vi "Read new data.vi"(7 "Scope":T1={"Config"={"VISA Resource"="", "Model"=enum."DPO 3012", "Timebase"=0.0, "Timeout (ms)"=0, "TAS"={"Vertical Range (V)"=0.0, "Vertical Offset (0.0 divs)"=0.0, "Bandwidth"=0, "Probe Attenuation (10.0)"=0.0, "Vertical Coupling"=0, "Impedance"=0, "Multiplication factor"=0.0, "Channel"=enum."Channel 1"}, "TPC"={"Vertical Range (V)"=0.0, "Vertical Offset (0.0 divs)"=0.0, "Bandwidth"=0, "Probe Attenuation (10.0)"=0.0, "Vertical Coupling"=0, "Impedance"=0, "Multiplication factor"=0.0, "Channel"=enum."Channel 1"}, "Trigger"={"Mode"=enum."Laser (TAS)", "Source "=enum."Channel 1", "PIA"={"Test LEDs"=FALSE, "LED line"="", "LED off (s)"=0.0, "LED on (s)"=0.0}, "Threshold (V)"=0.0004}}, "Indicators"={"Setup"={"Final number of points"=0.0, "Pretrigger points"=0.0, "Number of readouts"=0, "Model"={"Acquisition Type"=0, "Record length (points)"=0, "Averages on scope"=0, "Average number of points"=0.0}}, "Timestamp of Data"=timestamp(0 s since 1904-01-01)}, "Data"={"TPC"={"Live data"={"t0"=timestamp(0 s since 1904-01-01), "dt"=1.0, "Y"=[]}, "Averaged data"={"t0"=timestamp(0 s since 1904-01-01), "dt"=1.0, "Y"=[]}, "Accumulated data"={"t0"=timestamp(0 s since 1904-01-01), "dt"=1.0, "Y"=[]}, "Final data"={"t0"=timestamp(0 s since 1904-01-01), "dt"=1.0, "Y"=[]}}, "TAS"={"Live data"={"t0"=timestamp(0 s since 1904-01-01), "dt"=1.0, "Y"=[]}, "Averaged data"={"t0"=timestamp(0 s since 1904-01-01), "dt"=1.0, "Y"=[]}, "Accumulated data"={"t0"=timestamp(0 s since 1904-01-01), "dt"=1.0, "Y"=[]}, "Final data"={"t0"=timestamp(0 s since 1904-01-01), "dt"=1.0, "Y"=[]}}, "Time arrays"={"Time array (decimated)"=[], "waveform"={"t0"=timestamp(0 s since 1904-01-01), "dt"=1.0, "Y"=[]}}}, "Test"={"Config"={"Amplification Factor"=2.0, "100% Reflectance Standard"=2.0, "Calculation Method"=enum."Reflectance", "Option to discard new data?"=FALSE, "Mode"=enum."Spectrum", "Number of Averages"=0, "B Test?"=FALSE}, "Indicators"={"DAQ Background Level (V)"=2.0, "A-Test Counter"=2, "B-Test Counter"=2, "Type"=enum."A-Test", "Scope Background Level (Amps)"=2.0, "TAS only?"=FALSE}}} {"Test"."Config"."Number of Averages" min=0; "Indicators"."Setup"."Model"."Record length (points)" items=["1000"=1, "10,000"=10, "100,000"=100, "1,000,000"=1000, "5,000,000"=5000, "10,000,000"=10000]; "Indicators"."Setup"."Model"."Acquisition Type" items=["Sample", "Peak Detect", "Hi Res", "Envelope", "Average"]; "Config"."Trigger"."Threshold (V)" format="%#_3f"; "Config"."TPC"."Impedance" items=["1M", "75", "50"]; "Config"."TPC"."Vertical Coupling" items=["AC", "DC", "Ground"]; "Config"."TPC"."Bandwidth" items=["FULL", "250 MHz", "150 MHz", "20 MHz"]; "Config"."TAS"."Impedance" items=["1M", "75", "50"]; "Config"."TAS"."Vertical Coupling" items=["AC", "DC", "Ground"]; "Config"."TAS"."Bandwidth" items=["FULL", "250 MHz", "150 MHz", "20 MHz"]; "Config"."Timebase" format="%^#_3e"}, 8 "error in (no error)":errorcluster) -> (0 "error out":errorcluster, 3 "Two channels read":bool=TRUE, 5 "Scope out":T1={"Config"={"VISA Resource"="", "Model"=enum."DPO 3012", "Timebase"=0.0, "Timeout (ms)"=0, "TAS"={"Vertical Range (V)"=0.0, "Vertical Offset (0.0 divs)"=0.0, "Bandwidth"=0, "Probe Attenuation (10.0)"=0.0, "Vertical Coupling"=0, "Impedance"=0, "Multiplication factor"=0.0, "Channel"=enum."Channel 1"}, "TPC"={"Vertical Range (V)"=0.0, "Vertical Offset (0.0 divs)"=0.0, "Bandwidth"=0, "Probe Attenuation (10.0)"=0.0, "Vertical Coupling"=0, "Impedance"=0, "Multiplication factor"=0.0, "Channel"=enum."Channel 1"}, "Trigger"={"Mode"=enum."Laser (TAS)", "Source "=enum."Channel 1", "PIA"={"Test LEDs"=FALSE, "LED line"="", "LED off (s)"=0.0, "LED on (s)"=0.0}, "Threshold (V)"=0.0004}}, "Indicators"={"Setup"={"Final number of points"=0.0, "Pretrigger points"=0.0, "Number of readouts"=0, "Model"={"Acquisition Type"=0, "Record length (points)"=0, "Averages on scope"=0, "Average number of points"=0.0}}, "Timestamp of Data"=timestamp(0 s since 1904-01-01)}, "Data"={"TPC"={"Live data"={"t0"=timestamp(0 s since 1904-01-01), "dt"=1.0, "Y"=[]}, "Averaged data"={"t0"=timestamp(0 s since 1904-01-01), "dt"=1.0, "Y"=[]}, "Accumulated data"={"t0"=timestamp(0 s since 1904-01-01), "dt"=1.0, "Y"=[]}, "Final data"={"t0"=timestamp(0 s since 1904-01-01), "dt"=1.0, "Y"=[]}}, "TAS"={"Live data"={"t0"=timestamp(0 s since 1904-01-01), "dt"=1.0, "Y"=[]}, "Averaged data"={"t0"=timestamp(0 s since 1904-01-01), "dt"=1.0, "Y"=[]}, "Accumulated data"={"t0"=timestamp(0 s since 1904-01-01), "dt"=1.0, "Y"=[]}, "Final data"={"t0"=timestamp(0 s since 1904-01-01), "dt"=1.0, "Y"=[]}}, "Time arrays"={"Time array (decimated)"=[], "waveform"={"t0"=timestamp(0 s since 1904-01-01), "dt"=1.0, "Y"=[]}}}, "Test"={"Config"={"Amplification Factor"=2.0, "100% Reflectance Standard"=2.0, "Calculation Method"=enum."Reflectance", "Option to discard new data?"=FALSE, "Mode"=enum."Spectrum", "Number of Averages"=0, "B Test?"=FALSE}, "Indicators"={"DAQ Background Level (V)"=2.0, "A-Test Counter"=2, "B-Test Counter"=2, "Type"=enum."A-Test", "Scope Background Level (Amps)"=2.0, "TAS only?"=FALSE}}} {"Test"."Config"."Number of Averages" min=0; "Indicators"."Setup"."Model"."Record length (points)" items=["1000"=1, "10,000"=10, "100,000"=100, "1,000,000"=1000, "5,000,000"=5000, "10,000,000"=10000]; "Indicators"."Setup"."Model"."Acquisition Type" items=["Sample", "Peak Detect", "Hi Res", "Envelope", "Average"]; "Config"."Trigger"."Threshold (V)" format="%#_3f"; "Config"."TPC"."Impedance" items=["1M", "75", "50"]; "Config"."TPC"."Vertical Coupling" items=["AC", "DC", "Ground"]; "Config"."TPC"."Bandwidth" items=["FULL", "250 MHz", "150 MHz", "20 MHz"]; "Config"."TAS"."Impedance" items=["1M", "75", "50"]; "Config"."TAS"."Vertical Coupling" items=["AC", "DC", "Ground"]; "Config"."TAS"."Bandwidth" items=["FULL", "250 MHz", "150 MHz", "20 MHz"]; "Config"."Timebase" format="%^#_3e"})   [LabVIEW 2017, in "Scope.lvlib"]
doc: "Acquires either two channels or one channel of data from the scope, \ndepending on the mode (B-test only acquires Ch1/TAS data) and the \nuser's TPC channel selection (if channel is \"None\", we shouldn't acquire \ndata from it)"
uses:
  Scope.lvlib
  Controls/Params.ctl
  Controls/Models.ctl
  Controls/TPC.ctl
  Controls/Channels.ctl
  Trigger/Controls/Params.ctl
  Trigger/Controls/Mode.ctl
  Trigger/Controls/Trigger channels.ctl
  Controls/Acquisition type.ctl
  Controls/Record length.ctl
  Controls/Data.ctl
  Controls/Channel data.ctl
  System Control/CTLs/Test params.ctl
  System Control/CTLs/Test Controls.ctl
  System Control/CTLs/Test indicators.ctl
  System Control/CTLs/Test Type.ctl
  <vilib>/Waveform/WDTOps.llb/WDT Index Channel DBL.vi
  <vilib>/Utility/error.llb/Error Cluster From Error Code.vi
  <vilib>/ErrorRing/Error Ring.xnode
  Third Party Drivers/Tektronix DPO MSO 2000 4000 Series/Tektronix DPO MSO 2000 4000 Series.lvlib
  Processing/Processing.lvlib
  Trigger/Trigger.lvlib
  System Control/Main controller.lvlib
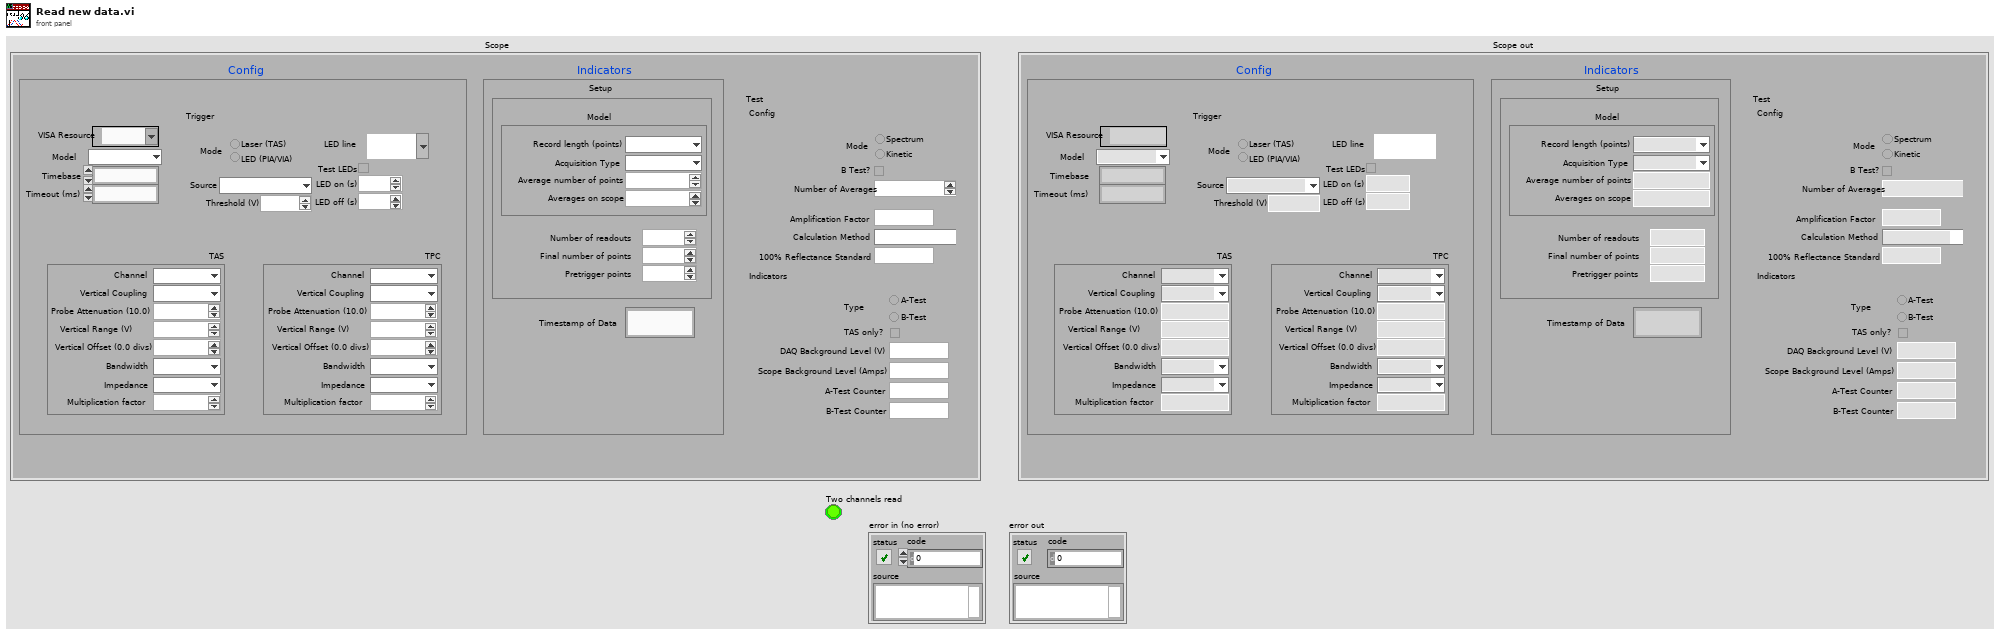
[diagram p1: front panel]
types:
  T1 = typedef "Scope.lvlib/Params.ctl" = cluster{"Config":cluster{"VISA Resource":refnum<visa-resource-name>, "Model":T2, "Timebase":dbl, "Timeout (ms)":u32, "TAS":T3, "TPC":T3, "Trigger":T5}, "Indicators":cluster{"Setup":cluster{"Final number of points":dbl, "Pretrigger points":dbl, "Number of readouts":i32, "Model":cluster{"Acquisition Type":T8, "Record length (points)":T9, "Averages on scope":i32, "Average number of points":dbl}}, "Timestamp of Data":timestamp}, "Data":T10, "Test":T12}
  T2 = typedef "Scope.lvlib/Models.ctl" = enum16{"DPO 3012", "DPO 2012B", "TDS 3012C"}
  T3 = typedef "Scope.lvlib/TPC.ctl" = cluster{"Vertical Range (V)":dbl, "Vertical Offset (0.0 divs)":dbl, "Bandwidth":i32, "Probe Attenuation (10.0)":dbl, "Vertical Coupling":u16, "Impedance":u16, "Multiplication factor":dbl, "Channel":T4}
  T4 = typedef "Scope.lvlib/Channels.ctl" = enum16{"Channel 1", "Channel 2", "Channel 3", "Channel 4", "Math", "Reference A", "Reference B", "Reference C", "Reference D", "B1", "B2", "None"}
  T5 = typedef "Scope.lvlib/Trigger.lvlib/Params.ctl" = cluster{"Mode":T6, "Source ":T7, "PIA":cluster{"Test LEDs":bool, "LED line":tag, "LED off (s)":dbl, "LED on (s)":dbl}, "Threshold (V)":dbl}
  T6 = typedef "Scope.lvlib/Trigger.lvlib/Mode.ctl" = enum32{"Laser (TAS)", "LED (PIA/VIA)"}
  T7 = typedef "Scope.lvlib/Trigger.lvlib/Trigger channels.ctl" = enum16{"Channel 1", "Channel 2", "Channel 3", "Channel 4", "AC Line", "Aux", "Digital Channel 0", "Digital Channel 1", "Digital Channel 2", "Digital Channel 3", "Digital Channel 4", "Digital Channel 5", "Digital Channel 6", "Digital Channel 7", "Digital Channel 8", "Digital Channel 9", "Digital Channel 10", "Digital Channel 11", "Digital Channel 12", "Digital Channel 13", "Digital Channel 14", "Digital Channel 15", "RF"}
  T8 = typedef "Scope.lvlib/Acquisition type.ctl" = u16
  T9 = typedef "Scope.lvlib/Record length.ctl" = u32
  T10 = typedef "Scope.lvlib/Data.ctl" = cluster{"TPC":T11, "TAS":T11, "Time arrays":cluster{"Time array (decimated)":dbl[], "waveform":waveform(dbl)}}
  T11 = typedef "Scope.lvlib/Channel data.ctl" = cluster{"Live data":waveform(dbl), "Averaged data":waveform(dbl), "Accumulated data":waveform(dbl), "Final data":waveform(dbl)}
  T12 = typedef "Main controller.lvlib/Test params.ctl" = cluster{"Config":T13, "Indicators":T14}
  T13 = typedef "Main controller.lvlib/Test Controls.ctl" = cluster{"Amplification Factor":dbl, "100% Reflectance Standard":dbl, "Calculation Method":enum16{"Reflectance", "Transmission", "Kubelka-Munk"}, "Option to discard new data?":bool, "Mode":enum32{"Spectrum", "Kinetic"}, "Number of Averages":i32, "B Test?":bool}
  T14 = typedef "Main controller.lvlib/Test indicators.ctl" = cluster{"DAQ Background Level (V)":dbl, "A-Test Counter":i32, "B-Test Counter":i32, "Type":T15, "Scope Background Level (Amps)":dbl, "TAS only?":bool}
  T15 = typedef "Main controller.lvlib/Test Type.ctl" = enum32{"A-Test", "B-Test"}
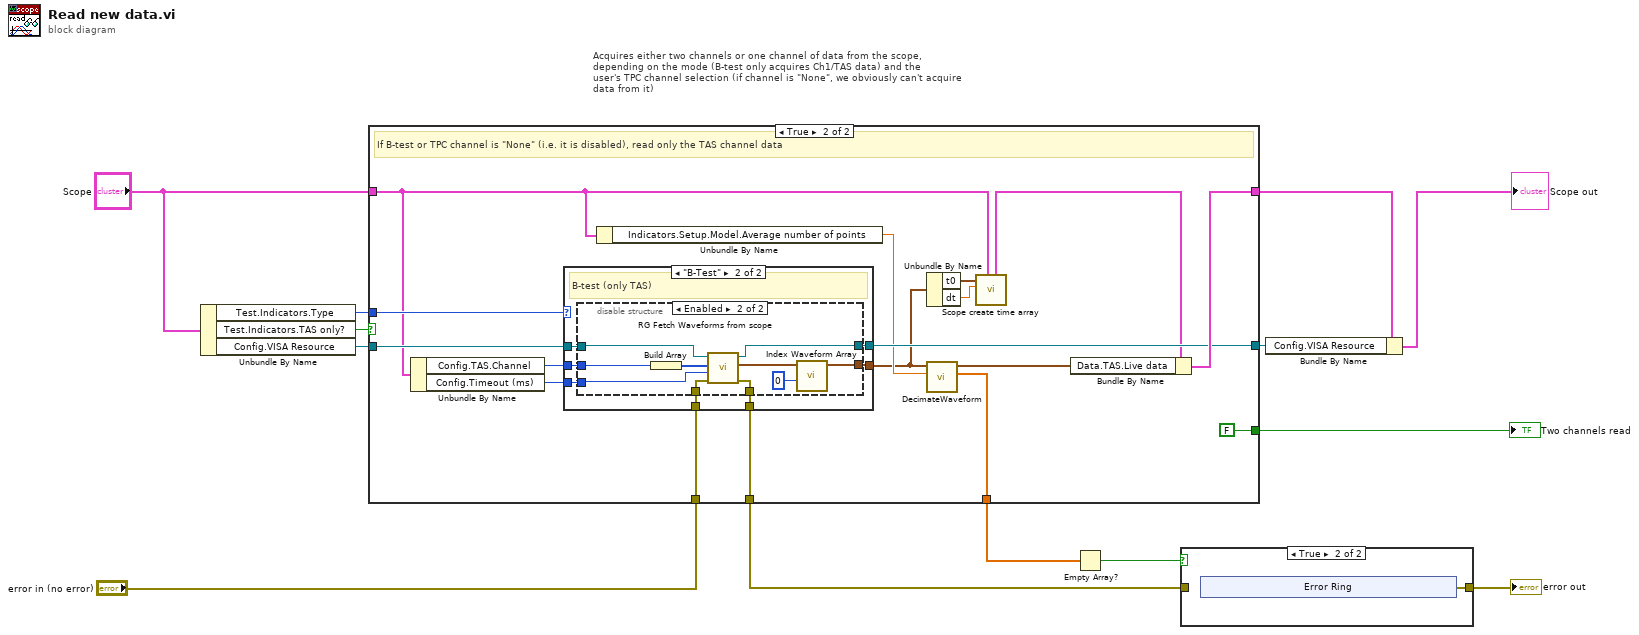
[diagram p0: block diagram]
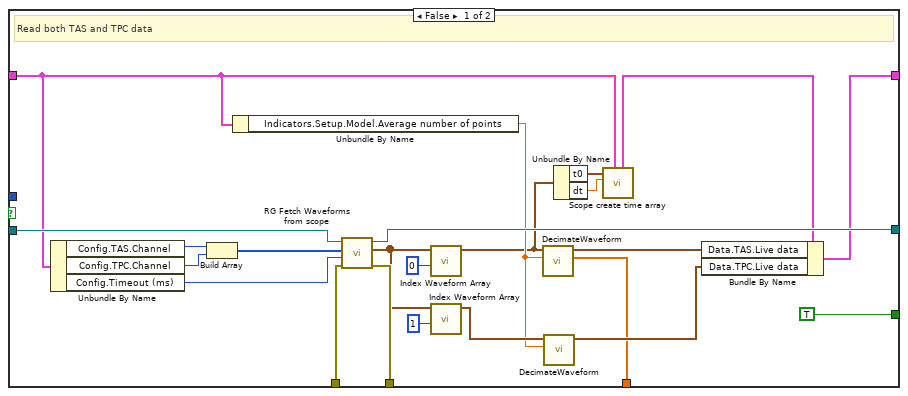
[diagram p2: hidden frame]
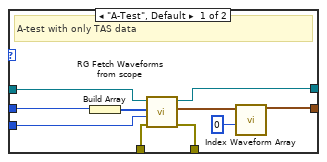
[diagram p3: hidden frame]
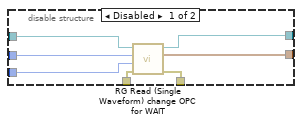
[diagram p4: hidden frame]
diagram:
  # "Acquires either two channels or one channel of data from the scope, \ndepending on the mode (B-test only acquires Ch1/TAS data) and the\nuser's TPC channel selection (if channel is \"None\", we obviously can't acquire data from it)"
  n1 = Unbundle By Name("Scope") -> ("Test.Indicators.Type"=w3:T15, "Test.Indicators.TAS only?"=w4:bool, "Config.VISA Resource"=w5:refnum<visa-resource-name>)
  n2 = case shown="True" w4 {
    tunnel: "error in (no error)" -> [w36 w50]
    tunnel: [w35 w49] -> w10
    tunnel: [w20 w42] -> w1
    tunnel: [w30 w51] -> w9
    tunnel: w5 -> [w29 w52]
    tunnel: "Scope" -> [w15 w41]
    tunnel: [w28 w53] -> w8
    tunnel: w3 -> [_ w46]
    tunnel: [TRUE FALSE] -> w6
    frame False {
      # "Read both TAS and TPC data"
      n3 = Unbundle By Name(w15) -> ("Config.TAS.Channel"=w33:T4, "Config.TPC.Channel"=w32:T4, "Config.Timeout (ms)"=w34:u32)
      n4 = Build Array(w33, w32) -> (w31:T4[])
      n5 = Unbundle By Name(w15) -> ("Indicators.Setup.Model.Average number of points"=w21:dbl)
      n6 = call "RG Fetch Waveforms from scope.vi"("error in (no error)"=w36, "Maximum Time (10000ms)"=w34, "Channels"=w31, "VISA resource name"=w29) -> ("error out"=w35:errorcluster, "Waveform Data"=w19:waveform(dbl)[], "VISA resource name out"=w30:refnum<visa-resource-name>)  [unwired: 5 in]
      n7 = call-poly <vilib>:"Index Waveform Array.vi"("index"=0, "waveform array"=w19) -> ("waveform"=w16:waveform(dbl))  [unwired: 8 in, 1 out]
      n8 = call-poly <vilib>:"Index Waveform Array.vi"("index"=1, "waveform array"=w19) -> ("waveform"=w23:waveform(dbl))  [unwired: 8 in, 1 out]
      n9 = call "DecimateWaveform.vi"("Decimating factor"=w21, "waveform in"=w16) -> ("Y"=w20:dbl[], "waveform out"=w22:waveform(dbl))  [unwired: 8 in]
      n10 = call "DecimateWaveform.vi"("Decimating factor"=w21, "waveform in"=w23) -> ("waveform out"=w24:waveform(dbl))  [unwired: 8 in, 1 out]
      n11 = Unbundle By Name(w16) -> ("t0"=w18:timestamp, "dt"=w17:dbl)
      n12 = call "Scope create time array.vi"("Scope"=w15, "dt"=w17, "t0"=w18) -> ("Scope Out"=w14:T1)  [unwired: 6 in, 2 out]
      n13 = Bundle By Name(cluster=w14, "Data.TAS.Live data"=w22, "Data.TPC.Live data"=w24) -> (w28:T1)
    }
    frame True {
      # "If B-test or TPC channel is \"None\" (i.e. it is disabled), read only the TAS channel data"
      n14 = Unbundle By Name(w41) -> ("Config.TAS.Channel"=w48:T4, "Config.Timeout (ms)"=w47:u32)
      n15 = case shown="\"B-Test\"" w46 {
        tunnel: w52 -> [w63 w67]
        tunnel: [w62 w68] -> w51
        tunnel: w50 -> [w60 w70]
        tunnel: [w59 w69] -> w49
        tunnel: w48 -> [w56 w66]
        tunnel: w47 -> [w61 w65]
        tunnel: [w57 w64] -> w39
        frame "A-Test", Default {
          # "A-test with only TAS data"
          n16 = Build Array(w56) -> (w55:T4[])
          n17 = call "RG Fetch Waveforms from scope.vi"("error in (no error)"=w60, "Maximum Time (10000ms)"=w61, "Channels"=w55, "VISA resource name"=w63) -> ("error out"=w59:errorcluster, "Waveform Data"=w54:waveform(dbl)[], "VISA resource name out"=w62:refnum<visa-resource-name>)  [unwired: 5 in]
          n18 = call-poly <vilib>:"Index Waveform Array.vi"("index"=0, "waveform array"=w54) -> ("waveform"=w57:waveform(dbl))  [unwired: 8 in, 1 out]
        }
        frame "B-Test" {
          # "B-test (only TAS)"
          n19 = disable-structure shown="Enabled" {
            disable-tunnel: w70 -> [w77 w79]
            disable-tunnel: [w76 w78] -> w69
            disable-tunnel: [w75 w84] -> w68
            disable-tunnel: w67 -> [w74 w83]
            disable-tunnel: w66 -> [w73 w81]
            disable-tunnel: w65 -> [w72 w82]
            disable-tunnel: [w71 w80] -> w64
            frame Disabled {
              n20 = call "RG Read (Single Waveform) change OPC for WAIT.vi"("error in (no error)"=w77, "Maximum Time (10000ms)"=w72, "Channel (0: Channel 1)"=w73, "VISA resource name"=w74) -> ("error out"=w76:errorcluster, "Waveform Graph"=w71:waveform(dbl), "VISA resource name out"=w75:refnum<visa-resource-name>)  [unwired: 5 in]
            }
            frame Enabled {
              n21 = Build Array(w81) -> (w87:T4[])
              n22 = call "RG Fetch Waveforms from scope.vi"("error in (no error)"=w79, "Maximum Time (10000ms)"=w82, "Channels"=w87, "VISA resource name"=w83) -> ("error out"=w78:errorcluster, "Waveform Data"=w86:waveform(dbl)[], "VISA resource name out"=w84:refnum<visa-resource-name>)  [unwired: 5 in]
              n23 = call-poly <vilib>:"Index Waveform Array.vi"("index"=0, "waveform array"=w86) -> ("waveform"=w80:waveform(dbl))  [unwired: 8 in, 1 out]
            }
          }
        }
      }
      n24 = Unbundle By Name(w41) -> ("Indicators.Setup.Model.Average number of points"=w43:dbl)
      n25 = Unbundle By Name(w39) -> ("t0"=w38:timestamp, "dt"=w37:dbl)
      n26 = call "DecimateWaveform.vi"("Decimating factor"=w43, "waveform in"=w39) -> ("Y"=w42:dbl[], "waveform out"=w44:waveform(dbl))  [unwired: 8 in]
      n27 = call "Scope create time array.vi"("Scope"=w41, "dt"=w37, "t0"=w38) -> ("Scope Out"=w40:T1)  [unwired: 6 in, 2 out]
      n28 = Bundle By Name(cluster=w40, "Data.TAS.Live data"=w44) -> (w53:T1)
    }
  }
  "Two channels read" <- w6
  n29 = Empty Array?(array=w1) -> (empty?=w12:bool)
  n30 = case shown="True" w12 {
    tunnel: [w88 w89] -> w11
    tunnel: w10 -> [w88 _]
    frame False {
    }
    frame True {
      n31 = xnode "Error Ring"() -> ("error out"=w89:errorcluster)
    }
  }
  "error out" <- w11
  n32 = Bundle By Name(cluster=w8, "Config.VISA Resource"=w9) -> (→"Scope out":T1)
